vi "Build Spectrums.vi"(1 "Waveforms":waveform(dbl)[](array[waveform])) -> (0 "Spectrums":waveform(dbl)[](array[waveform]))   [LabVIEW 2020]
uses:
  <vilib>/Analysis/4window.llb/windowTd.ctl
  <vilib>/measure/maspectr.llb/FFT Spectrum (Mag-Phase) for 1 Chan.vi
  <vilib>/measure/NI_MAPro.lvlib
  <vilib>/Analysis/NI_AALPro.lvlib
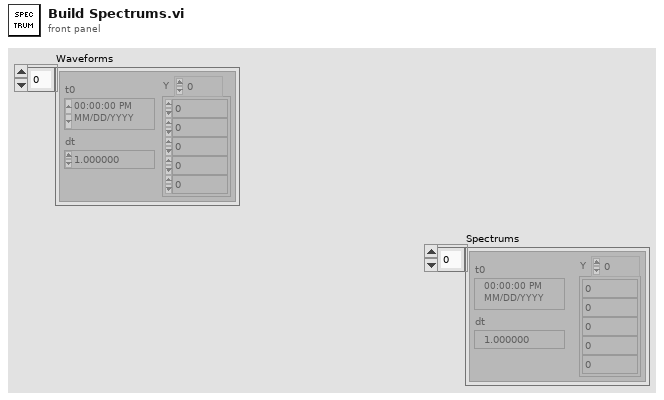
[diagram p1: front panel]
types:
  T1 = cluster{"dB On (F)":bool, "unwrap phase (F)":bool, "convert to degree (F)":bool}
  T2 = cluster{"averaging mode":enum16{"No averaging", "Vector averaging", "RMS averaging", "Peak hold"}, "weighting mode":enum16{"Linear", "Exponential"}, "number of averages":u32}
  T3 = typedef "NI_AALPro.lvlib/windowTd.ctl" = u32
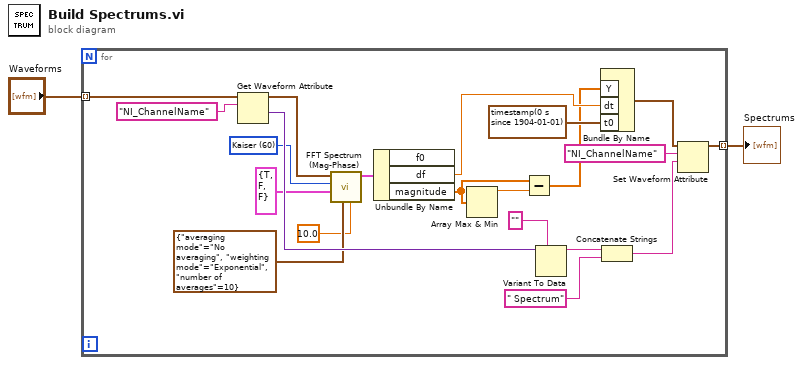
[diagram p0: block diagram]
diagram:
  n1 = for {
    tunnel: "Waveforms" -> [w23] mode=indexing
    tunnel: [w14] -> w1 mode=indexing
    w8 = T3 60 items=["Rectangle"=0, "Hanning"=1, "Hamming"=2, "Blackman-Harris"=3, "Exact Blackman"=4, "Blackman"=5, "Flat Top"=6, "4 Term B-Harris "=7, "7 Term B-Harris"=8, "Low Sidelobe"=9, "Blackman Nuttall"=11, "Triangle"=30, "Bartlett-Hanning"=31, "Bohman"=32, "Parzen"=33, "Welch"=34, "Kaiser"=60, "Dolph-Chebyshev"=61, "Gaussian"=62] ("window")
    n2 = Get Waveform Attribute(6:"NI_ChannelName" ("name"), 7:w23) -> (1:w21:variant, 3:w10:waveform(dbl))  [unwired: 2 in, 2 out]
    n3 = call-poly <vilib>:"FFT Spectrum (Mag-Phase).vi"("window parameter"=10.0, "averaging parameters"=T2 {"averaging mode"=enum."No averaging", "weighting mode"=enum."Exponential", "number of averages"=10}, "view"=T1 {"dB On (F)"=TRUE, "unwrap phase (F)"=FALSE, "convert to degree (F)"=FALSE}, "window"=w8, "time signal"=w10) -> ("magnitude"=w6:cluster{"f0":dbl, "df":dbl, "magnitude":dbl[]})  [unwired: 2 in, 4 out]
    n4 = Unbundle By Name(w6) -> ("df"=w11:dbl, "magnitude"=w5:dbl[])  [unwired: 1 out]
    n5 = Array Max & Min(array=w5) -> (max value=w4:dbl)  [unwired: 3 out]
    n6 = Subtract(x=w5, y=w4) -> (x-y=w3:dbl[])
    n7 = Variant To Data(type="" ("name"), Variant=w21) -> (data=w19:string)  [unwired: 1 in, 1 out]
    n8 = Bundle By Name("Y"=w3, "dt"=w11, "t0"=timestamp(0 s since 1904-01-01)) -> (w17:waveform(dbl))  [unwired: 1 in]
    n9 = Concatenate Strings(w19, " Spectrum" ("string")) -> (w15:string)
    n10 = Set Waveform Attribute(5:w15, 6:"NI_ChannelName" ("name"), 7:w17) -> (3:w14:waveform(dbl))  [unwired: 1 in, 2 out]
  }
  "Spectrums" <- w1
